vi "Pulse Messaging.vi"(8 "error in":errorcluster, 9 "Value":bool, 10 "Channel Name":string, 11 "DIG_IO in":refnum<class "DIG_IO.lvclass">) -> (0 "error out":errorcluster, 3 "DIG_IO out":refnum<class "DIG_IO.lvclass">)   [LabVIEW 2019, in "DIG_IO.lvlib" / "DIG_IO.lvclass"]
uses:
  Library/DIG_IO.lvclass
  C:/Users/Public/Documents/Development/builds/Engine/Engine.lvlibp/Project/Engine.lvclass
  DIG_IO Messages/Set by Name Msg/Set by Name Msg.lvclass
  C:/Users/Public/Documents/Development/builds/Engine/Actor Framework.lvlibp/1abvi3w/vi.lib/ActorFramework/Message/Message.lvclass
  DIG_IO Messages/Set by Name Msg/Set by Name Msg.lvclass/Set by Name Msg.ctl
  Accessors/Read Pulse Width.vi
  builds/Engine/Engine.lvlibp/Accessors/Read Self Q.vi
  builds/Engine/Actor Framework.lvlibp/1abvi3w/vi.lib/ActorFramework/Message Enqueuer/Enqueue.vi
  DIG_IO Messages/Set by Name Msg/SetAttributes.vi
  builds/Engine/Actor Framework.lvlibp/1abvi3w/vi.lib/ActorFramework/Message Enqueuer/Message Enqueuer.lvclass
  builds/Engine/Actor Framework.lvlibp
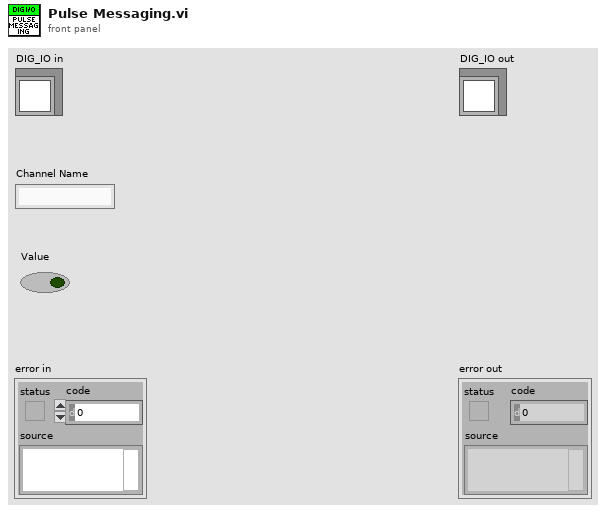
[diagram p1: front panel]
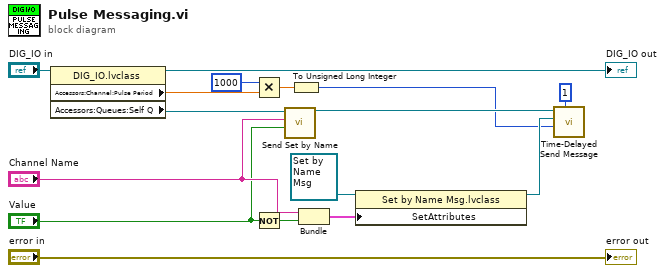
[diagram p0: block diagram]
diagram:
  n1 = property class="DIG_IO.lvclass"(reference="DIG_IO in") -> (reference out=→"DIG_IO out":refnum<class "DIG_IO.lvclass">, "Accessors:Channel:Pulse Period"=w4:dbl, "Accessors:Queues:Self Q"=w15:refnum<class "Message Enqueuer.lvclass">)  [unwired: 1 in, 1 out]
  n2 = Multiply(x=u32 1000 ("y"), y=w4) -> (x*y=w2:dbl)
  n3 = Not(x="Value") -> (.not. x?=w5:bool)
  n4 = call "Send Set by Name.vi"("Value"="Value", "Channel Name"="Channel Name", "Message Enqueuer"=w15) -> ("Message Enqueuer out"=w14:refnum<class "Message Enqueuer.lvclass">)  [unwired: 7 in, 1 out]
  n5 = To Unsigned Long Integer(number=w2) -> (unsigned 32bit integer=w1:u32)
  n6 = Bundle("Channel Name"="Channel Name", w5) -> (w8:cluster{"Channel Name":string, bool})  [unwired: 1 in]
  n7 = property class="Set by Name Msg.lvclass"(reference=refnum<class "Set by Name Msg.lvclass"> refnum ("DIG_IO.lvlib:Set by Name Msg.lvclass"), "SetAttributes"=w8) -> (reference out=w11:refnum<class "Set by Name Msg.lvclass">)  [unwired: 1 in, 1 out]
  n8 = call "Time-Delayed Send Message.vi"("# Copies (0 = infinite repeat)"=u32 1, "Milliseconds To Wait"=w1, "Message"=w11, "Message Enqueuer"=w14) -> ()  [unwired: 6 in, 2 out]
  "error out" <- "error in"
